vi "Obtain Queue.vi"(7 "Q Name":string, 8 "error in":errorcluster, 10 "Q element data type":variant, 11 "QueueMessageTransport in":refnum<class "QueueMessageTransport.lvclass">) -> (0 "error out":errorcluster, 3 "QueueMessageTransport out":refnum<class "QueueMessageTransport.lvclass">)   [LabVIEW 2016, in "QueueMessageTransport.lvclass"]
doc: "This public method creates a Queue reference\n\n**Author: Stas Legedza"
uses:
  QueueMessageTransport.lvclass
  QueueMessageTransport.lvclass/QueueMessageTransport.ctl
panel:
  # "INPUTS"
  # "OUTPUTS"
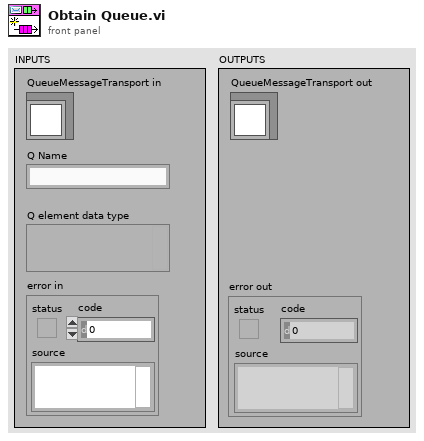
[diagram p1: front panel]
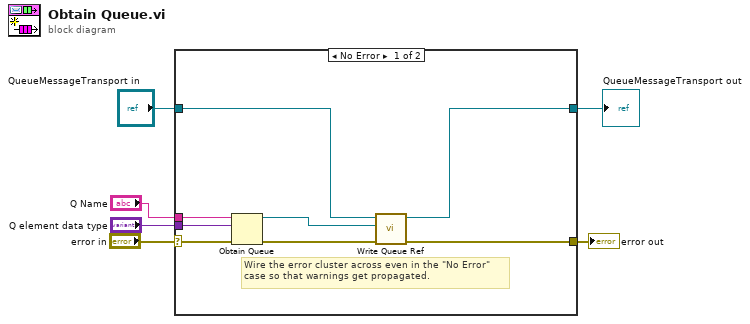
[diagram p0: block diagram]
diagram:
  n1 = case shown="No Error" "error in" {
    selector: "error in" -> [w12 w16]
    tunnel: [w11 w16] -> w5
    tunnel: [w7 w15] -> w3
    tunnel: "QueueMessageTransport in" -> [w10 w15]
    tunnel: "Q Name" -> [w14 _]
    tunnel: "Q element data type" -> [w13 _]
    frame No Error {
      # "Wire the error cluster across even in the \"No Error\"\ncase so that warnings get propagated."
      n2 = Obtain Queue(name (unnamed)=w14, element data type=w13, error in (no error)=w12) -> (queue out=w8:refnum<queue>, error out=w9:errorcluster)  [unwired: 2 in, 1 out]
      n3 = call "Write Queue Ref.vi"("error in"=w9, "Queue Ref"=w8, "QueueMessageTransport in"=w10) -> ("error out"=w11:errorcluster, "QueueMessageTransport out"=w7:refnum<class "QueueMessageTransport.lvclass">)  [unwired: 7 in]
    }
    frame Error {
    }
  }
  "error out" <- w5
  "QueueMessageTransport out" <- w3
